vi "data logger UI.vi"() -> ()   [LabVIEW 2020]
panel:
  in  "VISA resource name":refnum<visa-resource-name>
  in  "Table Control":string[][](table)
  out "Humidity":dbl(graph)
  out "Temp":dbl(graph)
  out "Humidity":dbl(knob) scale=0.0..100.0
  out "Thermometer":dbl(slide) scale=0.0..100.0
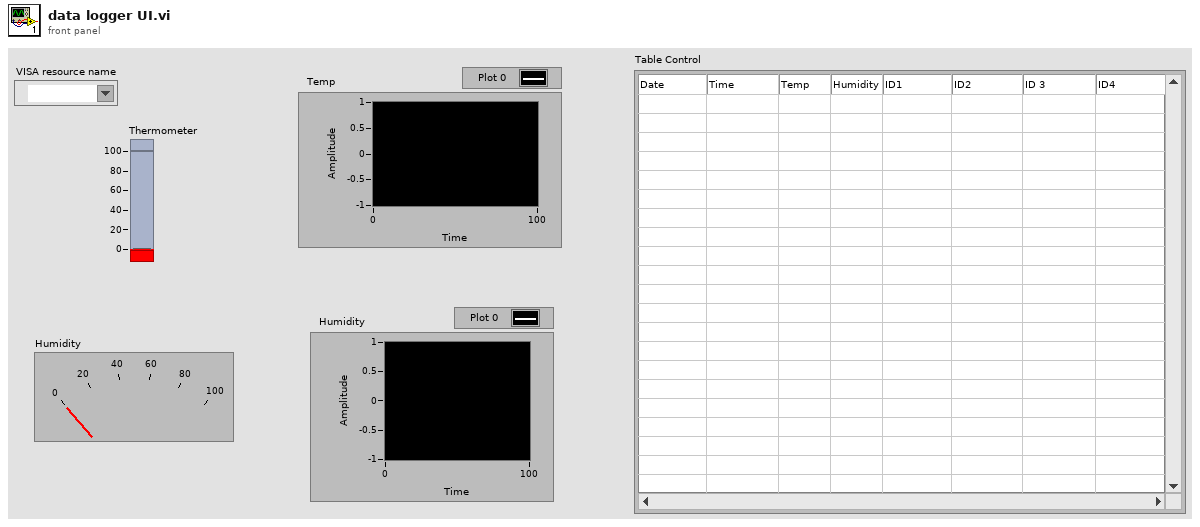
[diagram p1: front panel]
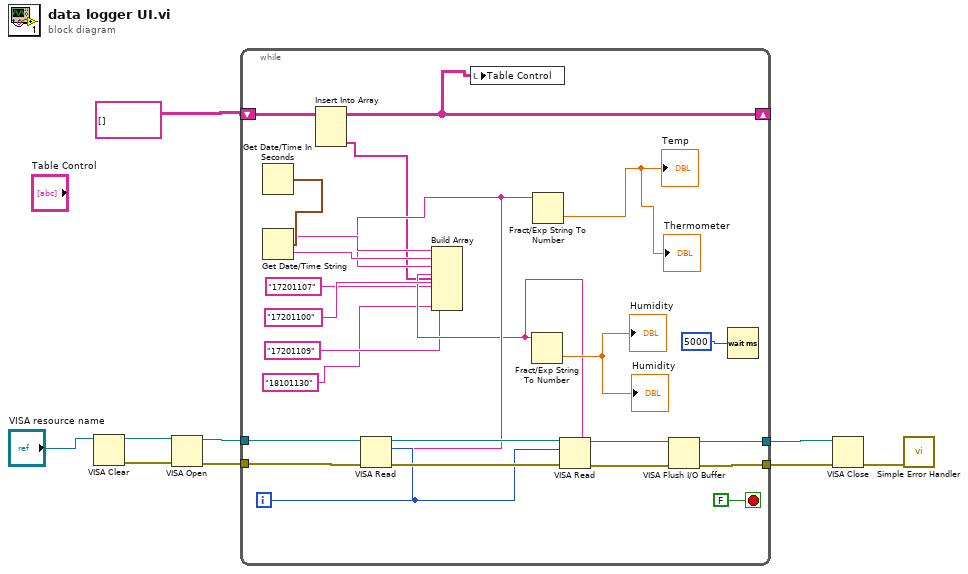
[diagram p0: block diagram]
diagram:
  n1 = VISA Clear(VISA resource name="VISA resource name") -> (VISA resource name out=w5:refnum<visa-resource-name>, error out=w6:errorcluster)  [unwired: 1 in]
  n2 = VISA Open(error in (no error)=w6, VISA resource name=w5) -> (VISA resource name=w4:refnum<visa-resource-name>, error out=w3:errorcluster)  [unwired: 3 in]
  n3 = while {
    tunnel: [w34] -> w8
    tunnel: [w33] -> w7
    tunnel: w4 -> [w27]
    tunnel: w3 -> [w26]
    shift-right: [w23] -> _
    shift-left: string[][] [] -> [w24]
    i -> [w28]
    stop <- FALSE stop-if-true
    n4 = Get Date/Time In Seconds() -> (seconds since 1Jan1904=w20:timestamp)
    n5 = Get Date/Time String(seconds (now)=w20) -> (date string=w19:string, time string=w18:string)  [unwired: 2 in]
    n6 = VISA Read(VISA resource name=w27, byte count=w28, error in (no error)=w26) -> (VISA resource name out=w30:refnum<visa-resource-name>, read buffer=w17:string, error out=w29:errorcluster)  [unwired: 1 out]
    n7 = Fract/Exp String To Number(string=w17) -> (number=→"Thermometer" →"Temp":dbl)  [unwired: 3 in, 1 out]
    n8 = VISA Read(VISA resource name=w30, byte count=w28, error in (no error)=w29) -> (VISA resource name out=w32:refnum<visa-resource-name>, read buffer=w14:string, error out=w31:errorcluster)  [unwired: 1 out]
    n9 = Build Array(w19, w18, w17, w14, "17201100" ("element"), "17201107" ("element"), "17201109" ("element"), "18101130" ("element")) -> (w13:string[])
    n10 = Insert Into Array(array=w24, new element=w13) -> (w23:string[][])  [unwired: 2 in]
    n11 = local write "Table Control"(w23) -> ()
    n12 = Fract/Exp String To Number(string=w14) -> (number=→"Humidity" →"Humidity":dbl)  [unwired: 3 in, 1 out]
    n13 = VISA Flush I/O Buffer(VISA resource name=w32, error in (no error)=w31) -> (VISA resource name out=w34:refnum<visa-resource-name>, error out=w33:errorcluster)  [unwired: 1 in]
    n14 = Wait (ms)(milliseconds to wait=u32 5000) -> ()  [unwired: 1 out]
  }
  n15 = VISA Close(VISA resource name=w8, error in (no error)=w7) -> (error out=w9:errorcluster)
  n16 = call <vilib>:"Simple Error Handler.vi"("error in (no error)"=w9) -> ()  [unwired: 4 in, 5 out]
